vi "closeHDF5.vi"(8 "error in (no error)":errorcluster, 11 "QuadraturePositionDecoder in":refnum<class "QuadraturePositionDecoder.lvclass">) -> (0 "error out":errorcluster, 3 "QuadraturePositionDecoder out":refnum<class "QuadraturePositionDecoder.lvclass">)   [LabVIEW 2014, in "QuadraturePositionDecoder.lvclass"]
uses:
  QuadraturePositionDecoder.lvclass
  QuadraturePositionDecoder.lvclass/QuadraturePositionDecoder.ctl
  private/HDF5Tools32/LabView/HDF5Tools.lvlib
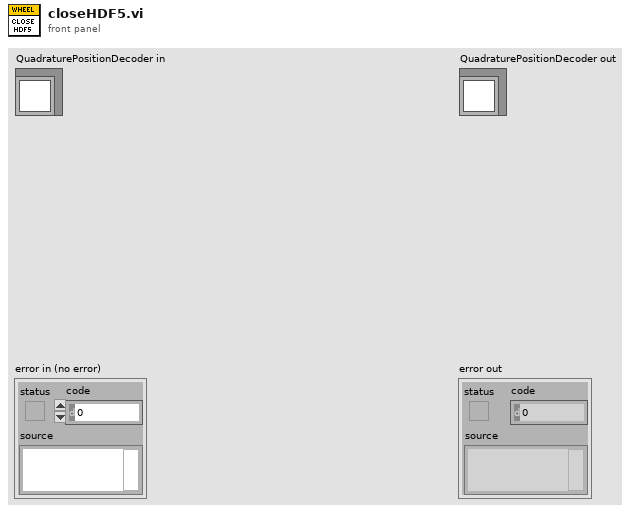
[diagram p1: front panel]
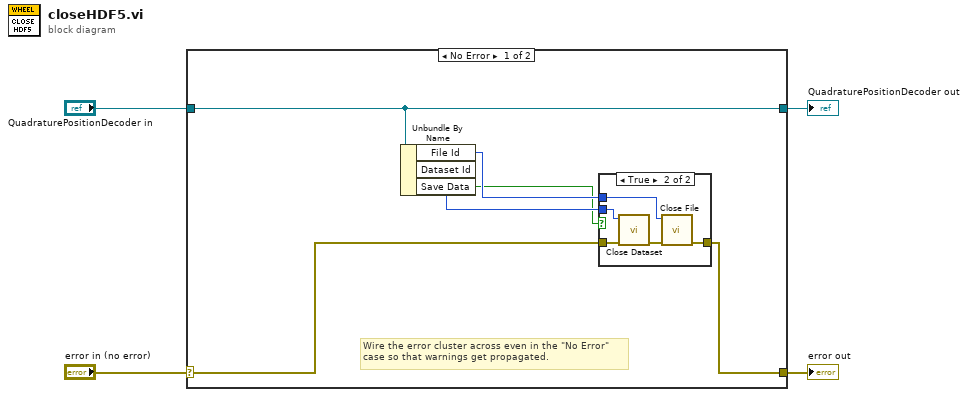
[diagram p0: block diagram]
diagram:
  n1 = case shown="No Error" "error in (no error)" {
    selector: "error in (no error)" -> [w7 w18]
    tunnel: [w6 w18] -> w3
    tunnel: [w10 w17] -> w1
    tunnel: "QuadraturePositionDecoder in" -> [w10 w17]
    frame No Error {
      # "Wire the error cluster across even in the \"No Error\"\ncase so that warnings get propagated."
      n2 = Unbundle By Name(w10) -> ("File Id"=w9:i32, "Dataset Id"=w8:i32, "Save Data"=w5:bool)
      n3 = case shown="True" w5 {
        tunnel: w8 -> [_ w15]
        tunnel: w9 -> [_ w14]
        tunnel: w7 -> [w11 w13]
        tunnel: [w11 w12] -> w6
        frame False {
        }
        frame True {
          n4 = call "Close Dataset.vi"("error in (no error)"=w13, "dataset_id"=w15) -> ("error out"=w16:errorcluster)  [unwired: 9 in]
          n5 = call "Close File.vi"("error in (no error)"=w16, "file_id"=w14) -> ("error out"=w12:errorcluster)  [unwired: 9 in]
        }
      }
    }
    frame Error {
    }
  }
  "error out" <- w3
  "QuadraturePositionDecoder out" <- w1
